vi "set Over Pressure Strategy.vi"(8 "error in (no error)":errorcluster, 10 "strategy":u32, 11 "pumpIndex":u32) -> (0 "error out":errorcluster, 3 "function return":i32)   [LabVIEW 2018, in "AsiaPumpInterface.lvlib"]
doc: "extern ASIAPUMP_INTERFACE_API BOOL setOverPressureStrategy( unsigned int pumpIndex ,\n unsigned int strategy );"
uses:
  <userlib>/AsiaPumpInterface/AsiaPumpInterface.lvlib
  <userlib>/AsiaPumpInterface/AsiaPumpInterface.dll
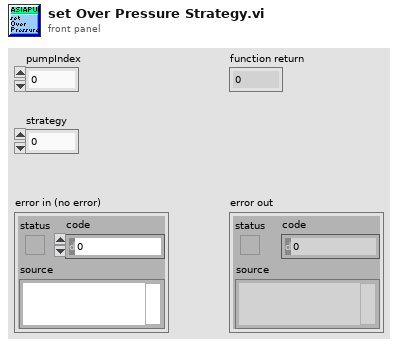
[diagram p1: front panel]
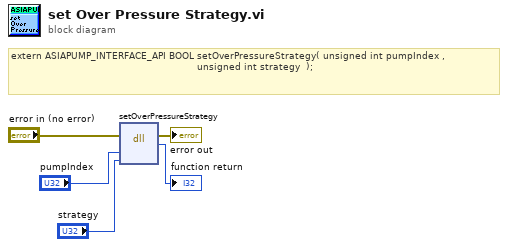
[diagram p0: block diagram]
diagram:
  # "extern ASIAPUMP_INTERFACE_API BOOL setOverPressureStrategy( unsigned int pumpIndex ,\n                                                              unsigned int strategy  );"
  n1 = dll-call lib="C:/Program Files (x86)/National Instruments/LabVIEW 2018/user.lib/AsiaPumpInterface/AsiaPumpInterface.*" fn="setOverPressureStrategy"(error in="error in (no error)", "pumpIndex"="pumpIndex", "strategy"="strategy") -> (error out=→"error out":errorcluster, →"function return":i32)  [unwired: 4 in, 1 out]
